vi "local.Commit Properties (Generic).vi"(0 "SLSC Local in":refnum<class "SLSC Interface.lvclass">, 5 "resources":string, 11 "error in (no error)":errorcluster) -> (4 "SLSC Local out":refnum<class "SLSC Interface.lvclass">, 15 "error out":errorcluster)   [LabVIEW 2016, in "SLSC Interface.lvclass"]
uses:
  SLSC Interface Class/SLSC Interface.lvclass
  SLSC Interface Class/Read session.vi
  SLSC Interface Class/Write session.vi
  <vilib>/SLSC/SLSC.lvlib
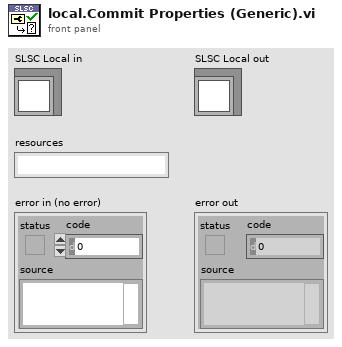
[diagram p1: front panel]
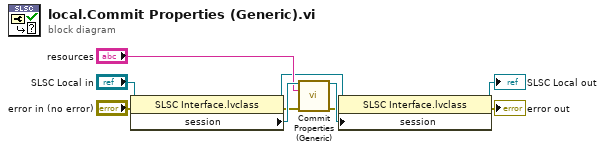
[diagram p0: block diagram]
diagram:
  n1 = property class="SLSC Interface.lvclass"(reference="SLSC Local in", error in="error in (no error)") -> (reference out=w6:refnum<class "SLSC Interface.lvclass">, error out=w3:errorcluster, "session"=w9:refnum<k21>)
  n2 = call <vilib>:"Commit Properties (Generic).vi"("session in"=w9, "resources"="resources", "error in (no error)"=w3) -> ("session out"=w8:refnum<k21>, "error out"=w2:errorcluster)  [unwired: 11 in]
  n3 = property class="SLSC Interface.lvclass"(reference=w6, error in=w2, "session"=w8) -> (reference out=→"SLSC Local out":refnum<class "SLSC Interface.lvclass">, error out=→"error out":errorcluster)
